vi "Lift Init.vi"   [LabVIEW 2014]
uses:
  Begin/Global RefNums.vi
  Begin/Global Variables.vi
types:
  T1 = typedef "WPI_SwitchDevRef.ctl" = cluster{"DevStatus":errorcluster, "DIO Channel":T2, "Controller":T3, "CntIndex":T4, "Normally Closed":bool}
  T2 = typedef "FPGA_DIOChannel.ctl" = enum8{"DIO 0", "DIO 1", "DIO 2", "DIO 3", "DIO 4", "DIO 5", "DIO 6", "DIO 7", "DIO 8", "DIO 9", "DIO MXP 0", "DIO MXP 1", "DIO MXP 2", "DIO MXP 3", "DIO MXP 4", "DIO MXP 5", "DIO MXP 6", "DIO MXP 7", "DIO MXP 8", "DIO MXP 9", "DIO MXP 10", "DIO MXP 11", "DIO MXP 12", "DIO MXP 13", "DIO MXP 14", "DIO MXP 15", "Invalid"}
  T3 = typedef "FPGA_TypedefDigitalModule.ctl" = enum16{"Controller 1"}
  T4 = typedef "FPGA_CounterCtrSystemIndex.ctl" = enum8{"Ctr 0", "Ctr 1", "Ctr 2", "Ctr 3", "Ctr 4", "Ctr 5", "Ctr 6", "Ctr 7", "Invalid"}
  T5 = typedef "WPI_MotorControlDeviceRef.ctl" = cluster{"DeviceStatus":errorcluster, "Type":T6, "PWM":cluster{"Controller":T3, "PWM Channel":T7, "DeadBand":T8}, "CAN":cluster{"Device Number":u8, "Control Mode":T9, "Semaphore":T10, "Max Vout":dbl, "TalonSRX Control Mode":T11}, "Invert":bool, "TransformRef":T12, "InvTransformRef":T12}
  T6 = typedef "WPI_MotorControlType.ctl" = enum16{"PWM", "CAN", "CANTalonSRX"}
  T7 = typedef "FPGA_DIOPWMChannel.ctl" = enum8{"PWM 0", "PWM 1", "PWM 2", "PWM 3", "PWM 4", "PWM 5", "PWM 6", "PWM 7", "PWM 8", "PWM 9", "PWM MXP 0", "PWM MXP 1", "PWM MXP 2", "PWM MXP 3", "PWM MXP 4", "PWM MXP 5", "PWM MXP 6", "PWM MXP 7", "PWM MXP 8", "PWM MXP 9", "Invalid"}
  T8 = typedef "WPI_PWMDeadband.ctl" = cluster{"Name":string, "maxPositivePwm":i32, "minPositivePwm":i32, "centerPwm":i32, "maxNegativePwm":i32, "minNegativePwm":i32, "angularRange":u16}
  T9 = typedef "WPI_CANJaguar_ControlMode.ctl" = enum8{"Percent VBus", "Current", "Speed", "Position", "Voltage"}
  T10 = typedef "Semaphore RefNum" = refnum<k1>
  T11 = typedef "WPI_CANTalonSRX_APIControlMode.ctl" = enum8{"Percent VBus", "Speed", "Position", "Slave", "Unchanged / Invalid"}
  T12 = typedef "WPI_PWMTransform_ConPane.ctl" = refnum<vi>
  T13 = typedef "WPI_EncoderDevRef.ctl" = cluster{"DevStatus":errorcluster, "EncoderIndex":T14, "CounterIndex":T4, "DistancePerCount":dbl, "Decoding Type":T15}
  T14 = typedef "FPGA_EncoderIdx.ctl" = enum8{"Enc 0", "Enc 1", "Enc 2", "Enc 3", "Enc 4", "Enc 5", "Enc 6", "Enc 7", "Invalid"}
  T15 = typedef "WPI_EncoderType.ctl" = enum16{"1x", "2x", "4x"}
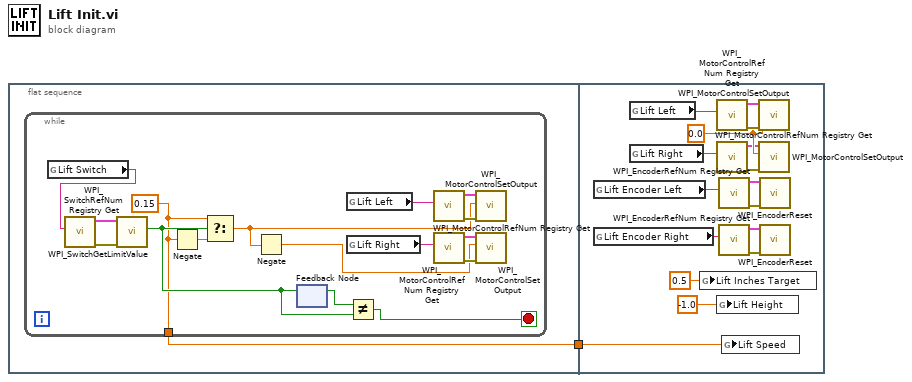
[diagram p0: block diagram]
diagram:
  n1 = flat-sequence {
    tunnel: [w2] -> w1
    tunnel: w1 -> [w21]
    frame #0 {
      n2 = while {
        tunnel: [w4] -> w2
        stop <- w5 stop-if-true
        w4 = 0.15 ("t")
        n3 = global read "Global RefNums.vi" "Lift Switch"() -> (w3:string)
        n4 = call <vilib>:"WPI_SwitchRefNum Registry Get.vi"("refnum name"=w3) -> ("error out"=w17:errorcluster, "SwitchDevRef"=w18:T1)  [unwired: 9 in]
        n5 = call <vilib>:"WPI_SwitchGetLimitValue.vi"("error in (no error)"=w17, "SwitchDevRef"=w18) -> ("Switch Pressed"=w6:bool)  [unwired: 7 in, 2 out]
        n6 = Negate(x=w4) -> (-x=w16:dbl)
        n7 = Select(t=w4, s=w6, f=w16) -> (s? t:f=w9:dbl)
        n8 = Negate(x=w9) -> (-x=w8:dbl)
        n9 = feedback-in #1(w6) -> ()
        n10 = feedback #1() -> (w7:bool)  [unwired: 1 in]
        n11 = global read "Global RefNums.vi" "Lift Left"() -> (w11:string)
        n12 = global read "Global RefNums.vi" "Lift Right"() -> (w10:string)
        n13 = Not Equal?(x=w7, y=w6) -> (x != y?=w5:bool)
        n14 = call <vilib>:"WPI_MotorControlRefNum Registry Get.vi"("refnum name"=w11) -> ("error out"=w15:errorcluster, "MotorControlDevRef"=w14:T5)  [unwired: 9 in]
        n15 = call <vilib>:"WPI_MotorControlRefNum Registry Get.vi"("refnum name"=w10) -> ("error out"=w12:errorcluster, "MotorControlDevRef"=w13:T5)  [unwired: 9 in]
        n16 = call <vilib>:"WPI_MotorControlSetOutput.vi"("error in (no error)"=w15, "Output"=w9, "MotorControlDevRef"=w14) -> ()  [unwired: 6 in, 3 out]
        n17 = call <vilib>:"WPI_MotorControlSetOutput.vi"("error in (no error)"=w12, "Output"=w8, "MotorControlDevRef"=w13) -> ()  [unwired: 6 in, 3 out]
      }
    }
    frame #1 {
      w27 = 0.0 ("Output")
      n18 = global read "Global RefNums.vi" "Lift Encoder Left"() -> (w32:string)
      n19 = global read "Global RefNums.vi" "Lift Encoder Right"() -> (w33:string)
      n20 = global read "Global RefNums.vi" "Lift Left"() -> (w23:string)
      n21 = global read "Global RefNums.vi" "Lift Right"() -> (w22:string)
      n22 = global write "Global Variables.vi" "Lift Inches Target"(0.5 ("Lift Inches Target")) -> ()
      n23 = call <vilib>:"WPI_MotorControlRefNum Registry Get.vi"("refnum name"=w23) -> ("error out"=w26:errorcluster, "MotorControlDevRef"=w20:T5)  [unwired: 9 in]
      n24 = call <vilib>:"WPI_MotorControlRefNum Registry Get.vi"("refnum name"=w22) -> ("error out"=w24:errorcluster, "MotorControlDevRef"=w25:T5)  [unwired: 9 in]
      n25 = global write "Global Variables.vi" "Lift Height"(-1.0 ("Lift Inches Target")) -> ()
      n26 = call <vilib>:"WPI_EncoderRefNum Registry Get.vi"("refnum name"=w32) -> ("error out"=w29:errorcluster, "EncoderDevRef"=w28:T13)  [unwired: 9 in]
      n27 = call <vilib>:"WPI_EncoderRefNum Registry Get.vi"("refnum name"=w33) -> ("error out"=w31:errorcluster, "EncoderDevRef"=w30:T13)  [unwired: 9 in]
      n28 = global write "Global Variables.vi" "Lift Speed"(w21) -> ()
      n29 = call <vilib>:"WPI_MotorControlSetOutput.vi"("error in (no error)"=w26, "Output"=w27, "MotorControlDevRef"=w20) -> ()  [unwired: 6 in, 3 out]
      n30 = call <vilib>:"WPI_MotorControlSetOutput.vi"("error in (no error)"=w24, "Output"=w27, "MotorControlDevRef"=w25) -> ()  [unwired: 6 in, 3 out]
      n31 = call <vilib>:"WPI_EncoderReset.vi"("error in (no error)"=w29, "EncoderDevRef"=w28) -> ()  [unwired: 8 in, 2 out]
      n32 = call <vilib>:"WPI_EncoderReset.vi"("error in (no error)"=w31, "EncoderDevRef"=w30) -> ()  [unwired: 8 in, 2 out]
    }
  }
